vi "FTW-Ether-CreateEndpoint.vi"(5 "Endpoint Type":T2, 7 "Message Transport Scheme":T1, 11 "error in":errorcluster) -> (4 "FTW Endpoint":refnum<class "FTW-Endpoint.lvclass">, 15 "error out":errorcluster)   [LabVIEW 2013, in "FTW-Ether.lvclass"]
uses:
  FTW-Ether.lvclass
  Endpoint/FTW-Endpoint.lvclass
  FTW-Ether-EndpointType.ctl
  FTW-Ether-MessageTransportScheme.ctl
  Notifier/FTW-Endpoint-Notifier.lvclass
panel:
  # "Inputs"
  # "Outputs"
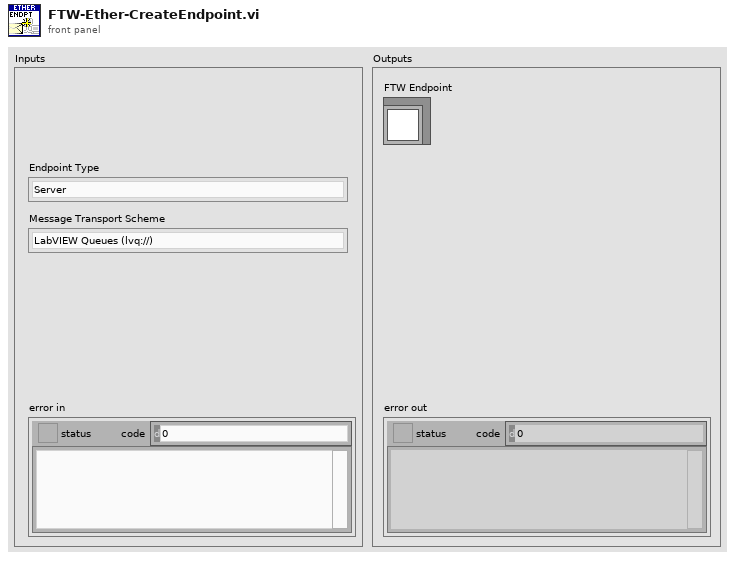
[diagram p1: front panel]
types:
  T1 = typedef "FTW-Ether.lvclass/FTW-Ether-MessageTransportScheme.ctl" = enum16{"LabVIEW Queues (lvq://)", "LabVIEW Notifiers (lvn://)", "LabVIEW Network Streams (lvns://)"}
  T2 = typedef "FTW-Ether.lvclass/FTW-Ether-EndpointType.ctl" = enum16{"Server", "Client", "Publisher", "Subscriber"}
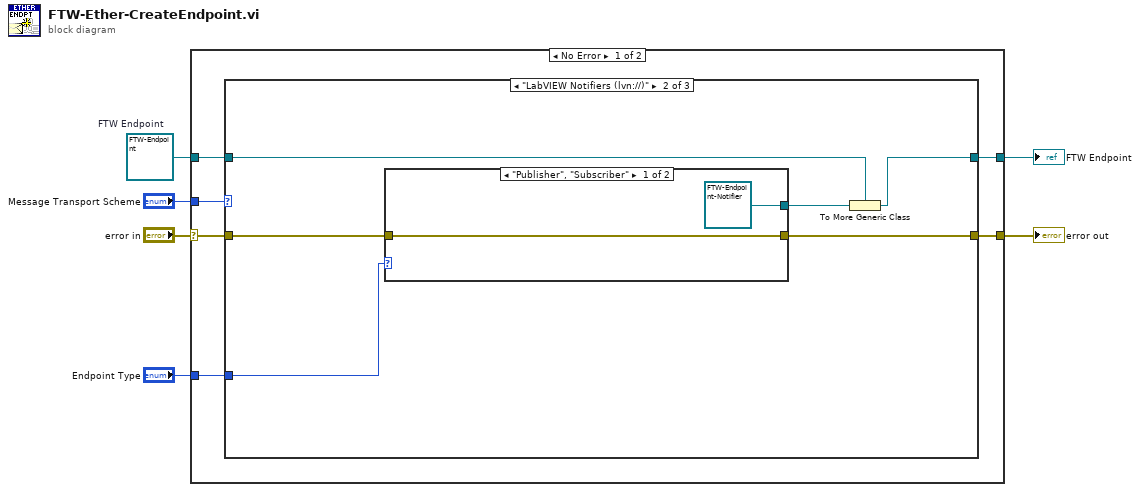
[diagram p0: block diagram]
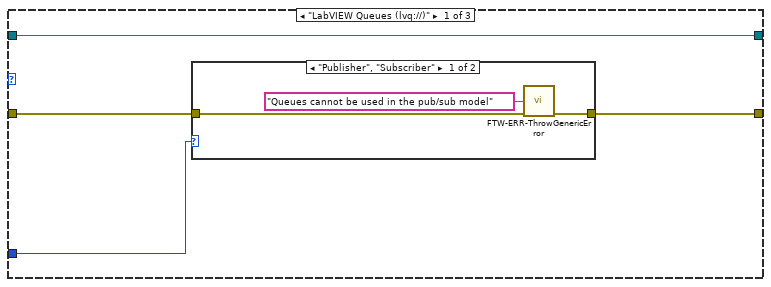
[diagram p2: hidden frame]
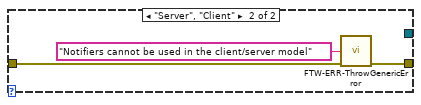
[diagram p4: hidden frame]
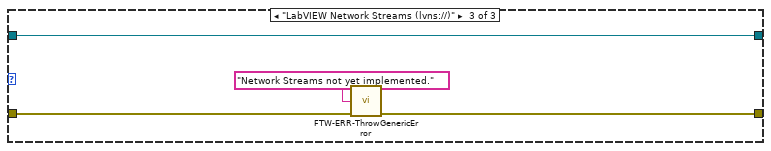
[diagram p5: hidden frame]
diagram:
  w1 = refnum<class "FTW-Endpoint.lvclass"> refnum  # FTW Endpoint
  n1 = case shown="No Error" "error in" {
    selector: "error in" -> [w9 w37]
    tunnel: [w12 w36] -> w6
    tunnel: [w11 w37] -> w5
    tunnel: "Message Transport Scheme" -> [w10 _]
    tunnel: "Endpoint Type" -> [w8 _]
    tunnel: w1 -> [w7 w36]
    frame No Error {
      n2 = case shown="\"LabVIEW Notifiers (lvn://)\"" w10 {
        tunnel: [w16 w22 w32] -> w12
        tunnel: [w15 w25 w33] -> w11
        tunnel: w9 -> [w14 w26 w34]
        tunnel: w8 -> [w13 w24 _]
        tunnel: w7 -> [w16 w23 w32]
        frame "LabVIEW Queues (lvq://)" {
          n3 = case shown="\"Publisher\", \"Subscriber\"" w13 {
            tunnel: w14 -> [w19 w20]
            tunnel: [w18 w20] -> w15
            frame "Publisher", "Subscriber" {
              n4 = call "FTW-ERR-ThrowGenericError.vi"("Error Message"="Queues cannot be used in the pub/sub model", "error in"=w19) -> ("error out"=w18:errorcluster)  [unwired: 13 in]
            }
            frame "Server", "Client" {
            }
          }
        }
        frame "LabVIEW Notifiers (lvn://)" {
          n5 = case shown="\"Publisher\", \"Subscriber\"" w24 {
            tunnel: w26 -> [w28 w31]
            tunnel: [w28 w30] -> w25
            tunnel: [refnum<class "FTW-Endpoint-Notifier.lvclass"> refnum ("Featherweight Actor:FTW Endpoint") _] -> w21
            frame "Publisher", "Subscriber" {
            }
            frame "Server", "Client" {
              n6 = call "FTW-ERR-ThrowGenericError.vi"("Error Message"="Notifiers cannot be used in the client/server model", "error in"=w31) -> ("error out"=w30:errorcluster)  [unwired: 13 in]
            }
          }
          n7 = To More Generic Class(target class=w23, reference=w21) -> (generic class reference=w22:refnum<class "FTW-Endpoint.lvclass">)
        }
        frame "LabVIEW Network Streams (lvns://)" {
          n8 = call "FTW-ERR-ThrowGenericError.vi"("Error Message"="Network Streams not yet implemented.", "error in"=w34) -> ("error out"=w33:errorcluster)  [unwired: 13 in]
        }
      }
    }
    frame Error {
    }
  }
  "error out" <- w5
  "FTW Endpoint" <- w6
